vi "DRAW_Trajectory_(offline).vi"(0 "Processing parameters":T1={"Defragment TDMS? (F)"=FALSE, "Start time (SW)"=timestamp(0 s since 1904-01-01), "Start time (HW)"=0, "Data filtering"={"Filter type"=enum."Savitzky-Golay", "Length"=41, "Order"=3}, "Mouse drawing parameters"={"Trace length, samples"=0, "Rainbow track"=FALSE, "Rainbow track is speed"=FALSE, "Bright mouse lineout"=FALSE, "Colors array"=[], "Pixels per mm"=0.0}, "Size of the image (480x480)"={"Numeric Control"=480.0, "Numeric Control"=480.0}, "Image ref. in"=refnum, "Calibration parameters"={"Timing calibration sw/hw"=1.0, "True FPS"=80.0, "True frame time, s"=0.0125, "Disp. calibration info"=[]}, "Pixel to zone"=[]} {"Calibration parameters"."True frame time, s" format="%.10g"; "Calibration parameters"."Disp. calibration info"."Speed, µl per ms" format="%.3g"; "Calibration parameters"."True FPS" format="%.10g"; "Calibration parameters"."Timing calibration sw/hw" format="%.10g"; "Data filtering"."Order" min=3 max=11 step=2; "Data filtering"."Length" min=5 max=301 step=2}, 5 "Animal coordinates and speed":T8, 7 "Track start, s":dbl=-1.0 format="%#_13g", 9 "Track finish, s":dbl=-1.0 format="%#_13g", 11 "Error In":errorcluster) -> (4 "Time-coded track overlay (array)":u32[][](array[numeric]), 6 "Speed-coded track overlay (array)":u32[][](array[numeric]), 8 "Plain track overlay pixmap":u32[][](array[numeric]) format="%x", 15 "Error Out":errorcluster)   [LabVIEW 2018, in "Tracker.lvlib"]
uses:
  Tracker.lvlib
  Controls/CTL_Animal_Coordinates_and_Speed_(arr).ctl
  Controls/CTL_Post-processing_params.ctl
  Controls/CTL_Filter_selector.ctl
  Controls/CTL_Mouse_Draw_Params.ctl
  <vilib>/vision/Image Controls.llb/IMAQ Image.ctl
  Controls/CTL_Calibration_parameters.ctl
  Controls/CTL_Dispenser_calibration_info.ctl
  Controls/CTL_Pixel_to_Zone_array.ctl
  <vilib>/Utility/miscctls.llb/LVBoundsTypeDef.ctl
  <resource>/objmgr/IMAQImage.rc
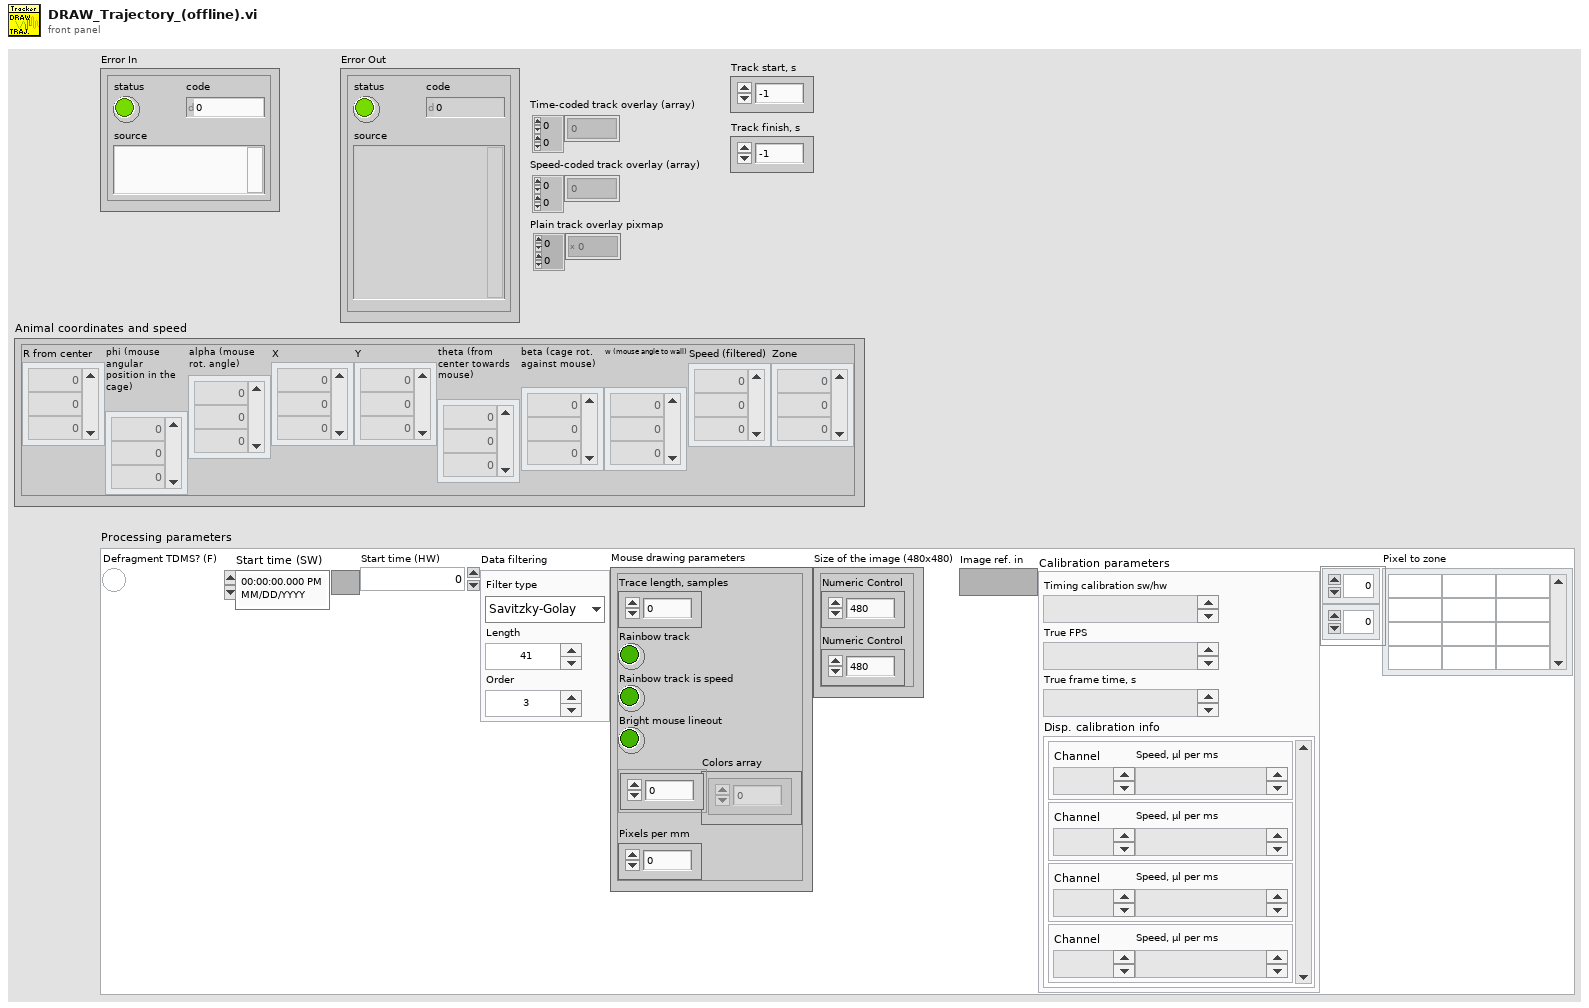
[diagram p1: front panel]
types:
  T1 = typedef "Tracker.lvlib/CTL_Post-processing_params.ctl" = cluster{"Defragment TDMS? (F)":bool, "Start time (SW)":timestamp, "Start time (HW)":u32, "Data filtering":T2, "Mouse drawing parameters":T3, "Size of the image (480x480)":cluster{"Numeric Control":dbl, "Numeric Control":dbl}, "Image ref. in":T4, "Calibration parameters":T5, "Pixel to zone":T7}
  T2 = typedef "Tracker.lvlib/CTL_Filter_selector.ctl" = cluster{"Filter type":enum16{"None", "Savitzky-Golay"}, "Length":i32, "Order":i32}
  T3 = typedef "Tracker.lvlib/CTL_Mouse_Draw_Params.ctl" = cluster{"Trace length, samples":u16, "Rainbow track":bool, "Rainbow track is speed":bool, "Bright mouse lineout":bool, "Colors array":u32[], "Pixels per mm":dbl}
  T4 = typedef "IMAQ Image.ctl" = refnum<image>
  T5 = typedef "Tracker.lvlib/CTL_Calibration_parameters.ctl" = cluster{"Timing calibration sw/hw":dbl, "True FPS":dbl, "True frame time, s":dbl, "Disp. calibration info":T6}
  T6 = typedef "Tracker.lvlib/CTL_Dispenser_calibration_info.ctl" = cluster{"Channel":u8, "Speed, µl per ms":dbl}[]
  T7 = typedef "Tracker.lvlib/CTL_Pixel_to_Zone_array.ctl" = i8[][]
  T8 = typedef "Tracker.lvlib/CTL_Animal_Coordinates_and_Speed_(arr).ctl" = cluster{"R from center":dbl[], "phi (mouse angular position in the cage)":dbl[], "alpha (mouse rot. angle)":dbl[], "X":dbl[], "Y":dbl[], "theta (from center towards mouse)":dbl[], "beta (cage rot. against mouse)":dbl[], "w (mouse angle to wall)":dbl[], "Speed (filtered)":dbl[], "Zone":i8[]}
  T9 = typedef "LVBoundsTypeDef.ctl" = cluster{"Width":u32, "Height":u32}
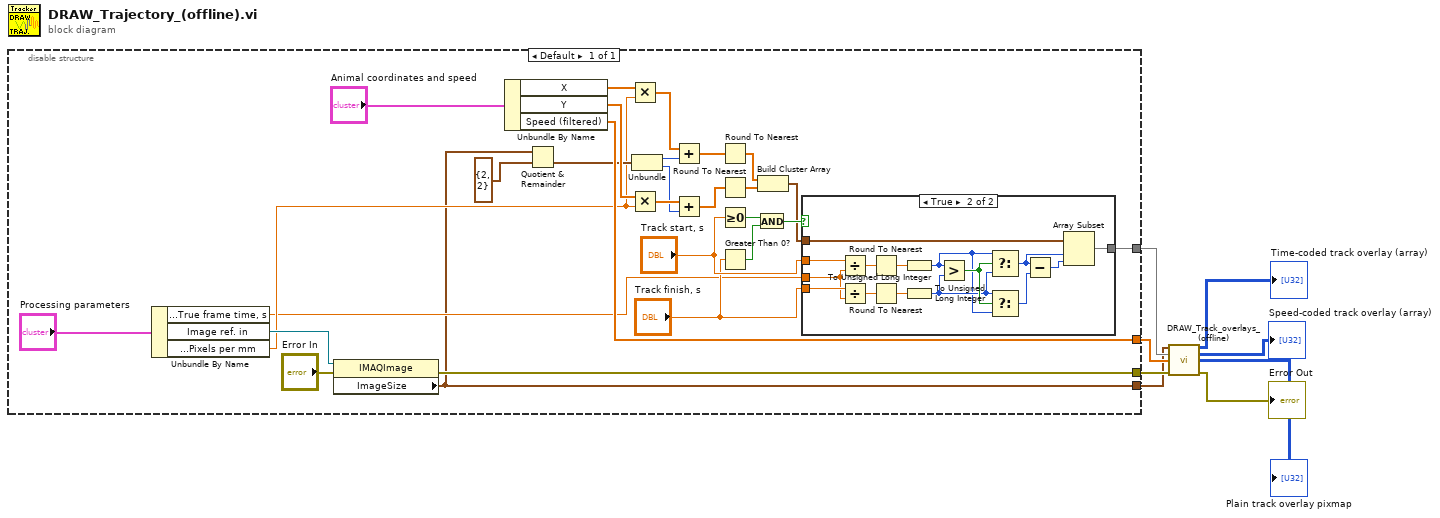
[diagram p0: block diagram]
diagram:
  n1 = disable-structure shown="Default" {
    disable-tunnel: [w31] -> w7
    disable-tunnel: [w11] -> w8
    disable-tunnel: [w10] -> w6
    disable-tunnel: [w9] -> w5
    frame Enabled {
      n2 = Unbundle By Name("Processing parameters") -> ("Calibration parameters.True frame time, s"=w13:dbl, "Image ref. in"=w20:T4, "Mouse drawing parameters.Pixels per mm"=w19:dbl)
      n3 = property class="IMAQImage"(reference=w20, error in="Error In") -> (error out=w10:errorcluster, "ImageSize"=w9:cluster{"x":i32, "y":i32})  [unwired: 1 out]
      n4 = Unbundle By Name("Animal coordinates and speed") -> ("X"=w34:dbl[], "Y"=w33:dbl[], "Speed (filtered)"=w31:dbl[])
      n5 = Quotient & Remainder(x=w9, y=T9 {"Width"=2, "Height"=2}) -> (floor(x/y)=w29:T9)  [unwired: 1 out]
      n6 = Multiply(x=w34, y=w19) -> (x*y=w36:dbl[])
      n7 = Multiply(x=w33, y=w19) -> (x*y=w35:dbl[])
      n8 = Unbundle(w29) -> ("Width"=w26:u32, "Height"=w25:u32)
      n9 = Add(x=w36, y=w26) -> (x+y=w28:dbl[])
      n10 = Add(x=w35, y=w25) -> (x+y=w27:dbl[])
      n11 = Round To Nearest(number=w28) -> (nearest integer value=w24:dbl[])
      n12 = Round To Nearest(number=w27) -> (nearest integer value=w23:dbl[])
      n13 = Greater Or Equal To 0?(x="Track start, s") -> (x >= 0?=w17:bool)
      n14 = Greater Than 0?(x="Track finish, s") -> (x > 0?=w18:bool)
      n15 = And(x=w17, y=w18) -> (x .and. y?=w16:bool)
      n16 = Build Cluster Array(w24, w23) -> (w12:cluster{dbl, dbl}[])
      n17 = case shown="True" w16 {
        tunnel: "Track start, s" -> [_ w52]
        tunnel: "Track finish, s" -> [_ w51]
        tunnel: w13 -> [_ w50]
        tunnel: w12 -> [w37 w45]
        tunnel: [w37 w44] -> w11
        frame False {
        }
        frame True {
          n18 = Divide(x=w52, y=w50) -> (x/y=w49:dbl)
          n19 = Divide(x=w51, y=w50) -> (x/y=w48:dbl)
          n20 = Round To Nearest(number=w49) -> (nearest integer value=w47:dbl)
          n21 = Round To Nearest(number=w48) -> (nearest integer value=w46:dbl)
          n22 = To Unsigned Long Integer(number=w47) -> (unsigned 32bit integer=w38:u32)
          n23 = To Unsigned Long Integer(number=w46) -> (unsigned 32bit integer=w39:u32)
          n24 = Greater?(x=w38, y=w39) -> (0:w42:bool)
          n25 = Select(t=w38, s=w42, f=w39) -> (s? t:f=w41:u32)
          n26 = Select(t=w39, s=w42, f=w38) -> (s? t:f=w40:u32)
          n27 = Subtract(x=w41, y=w40) -> (x-y=w43:u32)
          n28 = Array Subset(array=w45, index=w41, length=w43) -> (w44:cluster{dbl, dbl}[])
        }
      }
    }
  }
  n29 = call "DRAW_Track_overlays_(offline).vi"("Image size"=w5, "Full track array"=w8, "Speed array"=w7, "Error In"=w6) -> ("Time-coded overlay pixmap"=→"Time-coded track overlay (array)":u32[][], "Speed-coded overlay pixmap"=→"Speed-coded track overlay (array)":u32[][], "Plain track overlay pixmap"=→"Plain track overlay pixmap":u32[][], "Error Out"=→"Error Out":errorcluster)  [unwired: 8 in]
